vi "AlliGator Plot Fit Parameter 2 vs Parameter 1.vi"(7 "Lifetime Graph refnum":refnum<vi>, 8 "error in (no error)":errorcluster, 9 "Fit Parameter 2":T1, 10 "Fit Parameter 1":T1, 11 "Data Value Reference in":refnum<data-value>) -> (0 "error out":errorcluster, 3 "Data Value Reference out":refnum<data-value>, 4 "Message":string)   [LabVIEW 2021, in "AlliGator Decay Fit Parameter Map.lvlib"]
doc: "Creates scatter plot of selected parameter vs intensity for all ROIs and sends it to the <B>Lifetime & Other Parameters Graph</B>."
uses:
  AlliGator Decay Fit Parameter Map.lvlib
  Internal Variables/AlliGator Internal Variables v2.ctl
  <vilib>/vision/Image Controls.llb/IMAQ Image.ctl
  Internal Variables/AlliGator Gate Image Set.ctl
  Files/AlliGator FLI Dataset Type.ctl
  Files/AlliGator Data Series Type.ctl
  Dual-Channel Datasets/AlliGator Dataset Channel.ctl
  Settings/AlliGator Gate Arithmetic.ctl
  Source Image/AlliGator Displayed Image.ctl
  Image/Named ROI Description.ctl
  Phasor Graph/AlliGator Decay Metadata v3.ctl
  Decay Analysis/Decay Preprocessing/AlliGator Decay Background Subtraction Info.ctl
  Decay Analysis/Decay Preprocessing/AlliGator Baseline Subtraction Method.ctl
  Graphs/XY Graph/XY Graph Plot Shift Parameters.ctl
  Graphs/XY Graph/XY Graph Plot Shift Method.ctl
  Decay Analysis/Decay Preprocessing/AlliGator Decay Extrapolation Parameters.ctl
  Phasor/Calibration Phasor (m, phi).ctl
  Phasor/Phasor Reference Series.ctl
  Phasor/Phasor Calibration Map v2.ctl
  Phasor/Phasor (g, s).ctl
  Phasor Graph/AlliGator Raw Phasor Plot Data v5.ctl
  Phasor/Phasor Standard Deviation Options.ctl
  Phasor Plot/AlliGator Phasor Multi-Harmonic Data.ctl
  Phasor/Phasor Harmonic Data.ctl
  AlliGator Decay Fit Options & Parameters v4.ctl
  Fits/IRF(X)PSED/Decay Fit Options v4.ctl
  Fits/Decay Convolution/Decay Model.ctl
  Fits/Residual Type.ctl
  Fits/IRF(X)PSED/Fit Weights Type v2.ctl
  Fits/Non-linear Fitting Method v2.ctl
  Fits/Fit Calculation Method.ctl
  Fits/Non-linear Fitting Algorithm.ctl
  Decay Analysis/Decay Fit/AlliGator Decay Fit Parameter Constraints 2.ctl
  Fits/IRF(X)PSED/Decay Fit Parameters In List.ctl
  Fits/IRF(X)PSED/MLE Baseline Offset Type.ctl
  Decay Analysis/Decay Preprocessing/AlliGator Decay Preprocessing Parameters.ctl
  Fits/IRF(X)PSED/Decay Fit Parameters & Derived Quantities List v2.ctl
  Fits/IRF(X)PSED/Decay Fit Result Constraint.ctl
  AlliGator Parameter Maps Data.ctl
  Graphs/LabVIEW Plot Interpolation.ctl
  Graphs/Plot Point Style.ctl
  <userlib>/_OpenG.lib/array/array.llb/Filter 1D Array with Scalar (DBL)__ogtk.vi
  <userlib>/_OpenG.lib/array/array.llb/Delete Elements from 1D Array (DBL)__ogtk.vi
  <vilib>/Utility/error.llb/Error Cluster From Error Code.vi
  <vilib>/ErrorRing/Error Ring.xnode
  Files/AlliGator Files.lvlib
  Graphs/XY Graph/XY Graph Add-Ons.lvlib
  Graphs/Graphs.lvlib
  Image/Image.lvlib
  <userlib>/_OpenG.lib/array/array.llb/openg_array.lvlib
  Phasor/Phasor.lvlib
  Decay Analysis/Decay Preprocessing/AlliGator Decay Preprocessing.lvlib
  Phasor Graph/AlliGator Phasor Graph.lvlib
  Phasor Plot/AlliGator Phasor Plot.lvlib
  Source Image/AlliGator Source Image.lvlib
  Fits/Fits.lvlib
  Internal Variables/AlliGator Internal Variables.lvlib
  Decay Analysis/Decay Fit/AlliGator Decay Fit.lvlib
  Settings/AlliGator Settings.lvlib
  Dual-Channel Datasets/AlliGator Dual-Channel Datasets.lvlib
panel:
  in  "ROI idx (2147483647: all ROIs)":i32=2147483647
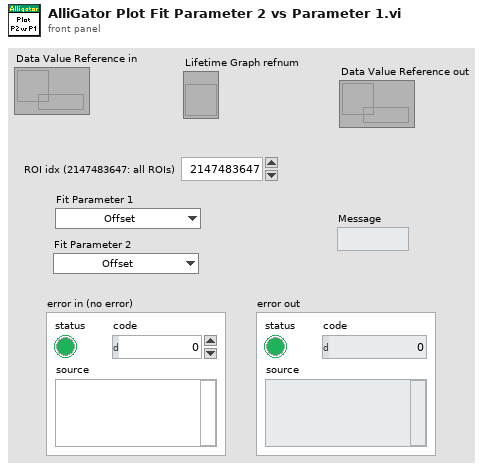
[diagram p1: front panel]
types:
  T1 = typedef "Fits.lvlib/Decay Fit Parameters & Derived Quantities List v2.ctl" = enum16{"Offset", "Baseline", "A_1", "tau_1", "A_2", "tau_2", "<tau>_a", "f1_a", "f2_a", "<tau>_i", "f1_i", "f2_i", "-", "R^2", "Chi^2"}
  T2 = typedef "Graphs.lvlib/Plot Point Style.ctl" = enum16{"not defined", "None", "Empty Circle", "Filled Circle", "Thick Circle", "Dotted Circle", "Empty Square", "Filled Square", "Thick Square", "Dotted Square", "Small Filled Square", "Dot", "Cross", "Tiny Cross", "Large X", "Small x", "Diamond", "Small Empty Square"}
  T3 = typedef "Graphs.lvlib/LabVIEW Plot Interpolation.ctl" = enum16{"Point (.)", "Stepwise Right (--.)", "Line + Point (\\. /)", "Stepwise Left (.--)", "Stepwise Centered (-.-)", "Stepwise Vertical (|.|)", "Line (-)", "Use Previous Plot's Style"}
  T4 = typedef "AlliGator Internal Variables.lvlib/AlliGator Internal Variables v2.ctl" = cluster{"----------------------------- Images -----------------------------":u8, "Displayed Image":T5, "White Light Image":T5, "Mask Image":T5, "ROI Mask Image":T5, "Current Dataset Images 1":T6, "Background Dataset Images 1":T6, "Current Dataset Images 2":T6, "Background Dataset Images 2":T6, "Current Dataset Arithmetic Images":T6, "Accumulated Dataset Images 1":T6, "Accumulated Dataset Images 2":T6, "Accumulated Dataset Arithmetic Images":T6, "----------------------------- File Paths -----------------------------":u8, "Phasor Plot Image":T5, "Decay Fit Parameter Map Image":T5, "Parameter Map Image":T5, "Single Data Point Path":path, "White Light Image Path":path, "Mask Image Path":path, "Time-Series Folder":path, "[Time-Series Paths]":path[], "----------------------------- FLI Dataset -----------------------------":u8, "Current Dataset":i32, "Single Dataset Type":T7, "Current Folder":string, "AlliGator Data Series Type":T8, "# Datasets":i32, "Dual-Channel Dataset":bool, "Selected Channel Name":string, "Dataset Channel":T9, "Channel Arithmetic":T10, "Dual-Channel Background Dataset":bool, "Background Channel":T9, "Dual-Channel Accumulated Dataset":bool, "Start Time":dbl, "[Time-Series Timestamps]":dbl[], "[Intensity Corrections]":dbl[], "Time Series Script":bool, "Type of Displayed Image":T11, "Gate Image Slide":u16, "# Gates":i32, "ROIs":T12[], "----------------------------- Decays -----------------------------":u8, "ROI Decay":cluster{"t Array":dbl[], "I Array":dbl[]}, "Valid Decay":bool, "Decay  Metadata":T14, "Reference Decay Plot Name":string, "Reference Decay":cluster{"t Array":dbl[], "I Array":dbl[]}, "Decay Shift Plot":cluster{"Time Stamps":dbl[], "Decay Shifts":dbl[]}, "[Decays Max Values]":sgl[], "[Decays Min Values]":sgl[], "----------------------------- Calibration -----------------------------":u8, "Calibration Phasor":T20, "Calibration Phasor Series":T21, "Phasor Calibration Map":T22, "Calibration Map MD5 Digest":string, "----------------------------- Phasor Graph -----------------------------":u8, "Last Raw Phasor":T23, "Last Calibrated Phasor":T23, "Last Calibrated Phasor SDV":T23, "Phasor Graph:Phasor Plot":cluster{"g Array":dbl[], "s Array":dbl[]}, "Phasor Graph:Phasor SDV Plot":cluster{"g Array":dbl[], "s Array":dbl[]}, "[Phasor Graph:Raw Phasor Plots]":T24[], "Phasor Plot locked to Ref 1":i32, "[Phasor Plot(s) locked to Ref 1]":i32[], "[Phasor Plot(s) locked to Ref 2]":i32[], "[Pixel Phasors]":T23[], "----------------------------- Phasor Plot -----------------------------":u8, "[[Sum Image]]":dbl[][], "[[CSG Phasors]]":csg[][], "[[Valid Pixel?]]":bool[][], "[[Phasor Ratios]]":dbl[][], "[[Average Lifetimes]]":dbl[][], "Amplitude Weighted Average Lifetime":bool, "I/m/phi Dataset":cluster{"I/m/phi Dataset?":bool, "Base Frequency":dbl[unit], "Harmonic Orders":u8[]}, "Multi Phasor Plot Data":T26, "----------------------------- Decay Fit Parameter Map -----------------------------":u8, "Decay Fit Options & Parameters":T28, "Fit Options: Decay Preprocessing Parameters":T39, "Fit Options: Reference Decay":cluster{"t Array":dbl[], "I Array":dbl[]}, "Is Full Image Parameters Map":bool, "Is Single-Pixels Parameters Map":bool, "NLSF Parameters Map X Resolution":i32, "NLSF Parameters Map Y Resolution":i32, "[Single Decay Fit Parameters]":dbl[], "Fit Model":T30, "[[Multiple Decays Fit Parameters]]":dbl[][], "[[Multiple Decays Fit Parameter SDVs]]":dbl[][], "[[IRFs]]":dbl[][], "[ROI Descriptors]":T13[], "IRF Array Time Axis":dbl[], "Decay Array Time Axis":dbl[], "[Decay Fit Parameter Names]":T1[], "[Decay Sum]":dbl[], "Array of Decay Fit Result Constraints":T40[], "Selected ROIs Array":bool[], "----------------------------- Parameter Maps -----------------------------":u8, "[Map Set Names]":string[], "[Parameter Maps]":T41[], "[[User-defined Quantities]]":dbl[][], "User-defined Quantity":string}
  T5 = typedef "IMAQ Image.ctl" = refnum<image>
  T6 = typedef "AlliGator Internal Variables.lvlib/AlliGator Gate Image Set.ctl" = cluster{"SGL Gate Images":T5[], "SGL Sum Image":T5, "SGL Max Image":T5, "SGL Min Image":T5}
  T7 = typedef "AlliGator Files.lvlib/AlliGator FLI Dataset Type.ctl" = enum16{"HDF5 FLI Dataset", "Gate Image Folder", ".sdt FLI Dataset (Becker & Hickl)", ".ptu FLI Dataset (PicoQuant)", "SS1 FLI Dataset", "SS2 FLI Dataset", "I/m/phi Dataset", ".bin FLI Dataset (PicoQuant Binned)", ".bin FLI Dataset (Piccolo Binned)", ".mat FLI Dataset"}
  T8 = typedef "AlliGator Files.lvlib/AlliGator Data Series Type.ctl" = enum16{"Not a Supported Series", "Gate Images Folder Series", "SwissSPAD 2 Dataset Series", "B&H FLI Dataset Series", "PicoQuant PTU FLI Dataset Series", "PicoQuant BIN FLI Dataset Series", "Piccolo hist BIN FLI Dataset Series", "HDF5 FLI Dataset Series"}
  T9 = typedef "AlliGator Dual-Channel Datasets.lvlib/AlliGator Dataset Channel.ctl" = enum16{"G2", "INT"}
  T10 = typedef "AlliGator Settings.lvlib/AlliGator Gate Arithmetic.ctl" = enum16{"None", "INT-G2", "G2/INT*<INT>", "(1 - G2/INT)*<INT>"}
  T11 = typedef "AlliGator Source Image.lvlib/AlliGator Displayed Image.ctl" = enum16{"Single Gate", "Sum of All Gates", "Max of All Gates", "Min of All Gates", "-", "White Ligth Image", "Mask Image"}
  T12 = typedef "Image.lvlib/Named ROI Description.ctl" = cluster{"ROI Descriptor":T13, "ROI Name":string, "Overlay Color":u32}
  T13 = typedef "ROI Descriptor" = cluster{"Global Rectangle":i32[], "Contours":cluster{"ID":enum32{"External", "Internal"}, "Type":u32, "Coordinates":i32[]}[]}
  T14 = typedef "AlliGator Phasor Graph.lvlib/AlliGator Decay Metadata v3.ctl" = cluster{"ROI Descriptor":T13, "ROI Center":cluster{"X":i32, "Y":i32}, "Decay Background Subtraction Info":T15, "Decay Reverted":bool, "Decay Smoothened":bool, "Decay Straightened":bool, "Fitted Tau (Decay Straightening)":dbl, "Decay Shift Parameters":T17, "Decay Shifted":bool, "Decay Extrapolated":bool, "Decay Extrapolation Parameters":T19, "Decay Normalized":bool, "Fold Decay":bool, "# Folds":u32}
  T15 = typedef "AlliGator Decay Preprocessing.lvlib/AlliGator Decay Background Subtraction Info.ctl" = cluster{"Laser Period":dbl[unit], "Gate Duration":dbl[unit], "Baseline Subtraction Method":T16, "Background Definition Range":cluster{"Min Gate":dbl[unit], "Max Gate":dbl[unit]}, "Total Intensity w/o Bkgd Subtraction":dbl, "Bkgd-subtracted Intensity (exp)":dbl, "# Data Points":i32, "Background/Gate":dbl, "Fitted Lifetime":dbl[unit], "Bkgd-subtracted Intensity (theo)":dbl}
  T16 = typedef "AlliGator Decay Preprocessing.lvlib/AlliGator Baseline Subtraction Method.ctl" = enum16{"Mean", "Min", "Square Gated Single-Exponential", "File", "Constant"}
  T17 = typedef "XY Graph Add-Ons.lvlib/XY Graph Plot Shift Parameters.ctl" = cluster{"Type":T18, "Shift":dbl[unit], "Threshold":dbl, "Rotate":bool}
  T18 = typedef "XY Graph Add-Ons.lvlib/XY Graph Plot Shift Method.ctl" = enum16{"Default", "CFD", "Threshold", "Cross-Correlation"}
  T19 = typedef "AlliGator Decay Preprocessing.lvlib/AlliGator Decay Extrapolation Parameters.ctl" = cluster{"Additional Points":u32, "Head Fraction":dbl, "Fitted Tau":dbl, "Use Periodicity":bool, "Use Cursors":bool, "Tail Fraction":dbl}
  T20 = typedef "Phasor.lvlib/Calibration Phasor (m, phi).ctl" = cluster{"m":dbl, "phi":dbl, "Phasor Frequency":dbl[unit], "Reference Lifetime":dbl[unit]}
  T21 = typedef "Phasor.lvlib/Phasor Reference Series.ctl" = cluster{"m Array":dbl[], "phi Array":dbl[], "Phasor Frequency":dbl[unit], "Calibration Lifetime":dbl[unit]}
  T22 = typedef "Phasor.lvlib/Phasor Calibration Map v2.ctl" = cluster{"Phasor Frequency":dbl[unit], "Calibration Lifetime":dbl[unit], "ROI Centers":cluster{"X":i32, "Y":i32}[], "ROI Descriptors":T13[], "Map Resolution X":i32, "Map Resolution Y":i32, "z Array":cdb[]}
  T23 = typedef "Phasor.lvlib/Phasor (g, s).ctl" = cluster{"g":dbl, "s":dbl}
  T24 = typedef "AlliGator Phasor Graph.lvlib/AlliGator Raw Phasor Plot Data v5.ctl" = cluster{"Phasor Plot Name":string, "Raw Phasor Plot":T23[], "Phasor Frequency":dbl[unit], "[Decay Metadata]":T14[], "Raw Phasor Plot SDV":T23[], "Phasor SDV Options":T25, "[Calibration Phasor]":T20[], "Intensity Array":dbl[]}
  T25 = typedef "Phasor.lvlib/Phasor Standard Deviation Options.ctl" = cluster{"Compute Estimated SDV":bool, "# Replicas":u32, "Use Estimated Average Phasor":bool}
  T26 = typedef "AlliGator Phasor Plot.lvlib/AlliGator Phasor Multi-Harmonic Data.ctl" = cluster{"Base Frequency":dbl[unit], "# Harmonics":u8, "Harmonic Orders":u8[], "Phasor Plot Settings Checksum":u64, "Phasor Harmonic Data Array":T27[]}
  T27 = typedef "Phasor.lvlib/Phasor Harmonic Data.ctl" = cluster{"Phasor Harmonic Name":string, "Phasor Plot Settings Checksum":u64, "Phasor Frequency":dbl[unit], "Base Frequency":dbl[unit], "Harmonic Order":u8, "Phasor Plot Parameters":string, "Phasor Array [[CSG]]":csg[][], "Dataset File Path":path}
  T28 = typedef "AlliGator Decay Fit Parameter Map.lvlib/AlliGator Decay Fit Options & Parameters v4.ctl" = cluster{"SYNC Period":dbl[unit], "Fit Options":T29, "Fit Parameter Constraints":T36[], "MLE Baseline Offset":dbl, "MLE Baseline Offset Type":T38}
  T29 = typedef "Fits.lvlib/Decay Fit Options v4.ctl" = cluster{"Show Fit Residuals":bool, "Fit Model":T30, "Residual Type":T31, "Max Decay Percentile":dbl, "Min Decay Percentile":dbl, "Show Full Decay":bool, "Weights":T32, "Fitting Method":T33, "Compute Parameter Uncertainties":bool, "Periodic Boundaries":bool, "Model Calculation":T34, "Period":dbl[unit], "Termination Criteria":cluster{"Max Iterations":i32, "Max Function Calls":i32, "Max Time":dbl[unit], "Function Tolerance":dbl, "Parameter Tolerance":dbl, "Gradient Tolerance":dbl, "Min Lambda":dbl, "Max Lambda":dbl, "Initial Tick Count":u32}, "Offset Resolution":dbl[unit], "Use Local IRF":bool, "Fitting Algorithm":T35, "Show Confidence Interval ":bool, "Confidence Level":dbl}
  T30 = typedef "Fits.lvlib/Decay Model.ctl" = enum16{"1-Exponential", "2-Exponentials"}
  T31 = typedef "Fits.lvlib/Residual Type.ctl" = enum16{"Standard", "Normalized", "Reduced"}
  T32 = typedef "Fits.lvlib/Fit Weights Type v2.ctl" = enum16{"Unweighted", "1/Variance (Neyman)", "1/Variance (Pearson)", "Best of All"}
  T33 = typedef "Fits.lvlib/Non-linear Fitting Method v2.ctl" = enum16{"Least Square", "Least Absolute Residual", "Bisquare", "MLE", "-", "Best of All"}
  T34 = typedef "Fits.lvlib/Fit Calculation Method.ctl" = enum16{"Simulation", "Convolution", "Integration"}
  T35 = typedef "Fits.lvlib/Non-linear Fitting Algorithm.ctl" = enum16{"Levenberg-Marquardt", "Trust-Region Dogleg"}
  T36 = typedef "AlliGator Decay Fit.lvlib/AlliGator Decay Fit Parameter Constraints 2.ctl" = cluster{"Fit Parameter":T37, "Min Value":dbl, "Max Value":dbl, "Global":bool, "Used":bool}
  T37 = typedef "Fits.lvlib/Decay Fit Parameters In List.ctl" = enum16{"Offset", "Baseline", "A_1", "tau_1", "A_2", "tau_2"}
  T38 = typedef "Fits.lvlib/MLE Baseline Offset Type.ctl" = enum32{"Absolute", "Percentage"}
  T39 = typedef "AlliGator Decay Preprocessing.lvlib/AlliGator Decay Preprocessing Parameters.ctl" = cluster{"Background Subtraction":bool, "Straighten Decay":bool, "Reverse Gates":bool, "1-Normalized Decay":bool, "Smoothen Decay":bool, "Smoothing Parameter":dbl, "Shift Decay":bool, "Decay Shift Parameters":T17, "Extrapolate Decay":bool, "Additional Points":u32, "Head Fraction":dbl, "Pixel-Normalize Decay":bool, "Use Periodicity":bool, "Use Cursors":bool, "Tail Fraction":dbl, "Use Decay Pre-Processing":bool, "Fold Decay":bool, "# Folds":u32, "[0-1]-Normalized Decay":bool}
  T40 = typedef "Fits.lvlib/Decay Fit Result Constraint.ctl" = cluster{"Fit Parameter":enum16{"Offset", "Baseline", "A_1", "tau_1", "A_2", "tau_2", "<tau>_a", "f1_a", "f2_a", "<tau>_i", "f1_i", "f2_i", "-", "R^2", "Chi^2", "Max Relative Residual", "<Residual ACF>", "Residual ACF SDV", "tau_2/tau_1"}, "Min Value":dbl, "Max Value":dbl, "Use Constraint":bool}
  T41 = typedef "AlliGator Decay Fit Parameter Map.lvlib/AlliGator Parameter Maps Data.ctl" = cluster{"Map Set Name":string, "[Parameter Names]":string[], "[[Parameters]]":dbl[][], "[[Parameter SDVs]]":dbl[][], "Decay Array Time Axis":dbl[], "[[IRFs]]":dbl[][], "IRF Array Time Axis":dbl[], "X Resolution":i32, "Y Resolution":i32, "Intensity Array":dbl[]}
  T42 = typedef "XY Graph Add-Ons.lvlib/XY Graph Refnum.ctl" = refnum<vi>
  T43 = cluster{"array w/ subset deleted":dbl[], "array w/ subset deleted":dbl[]}
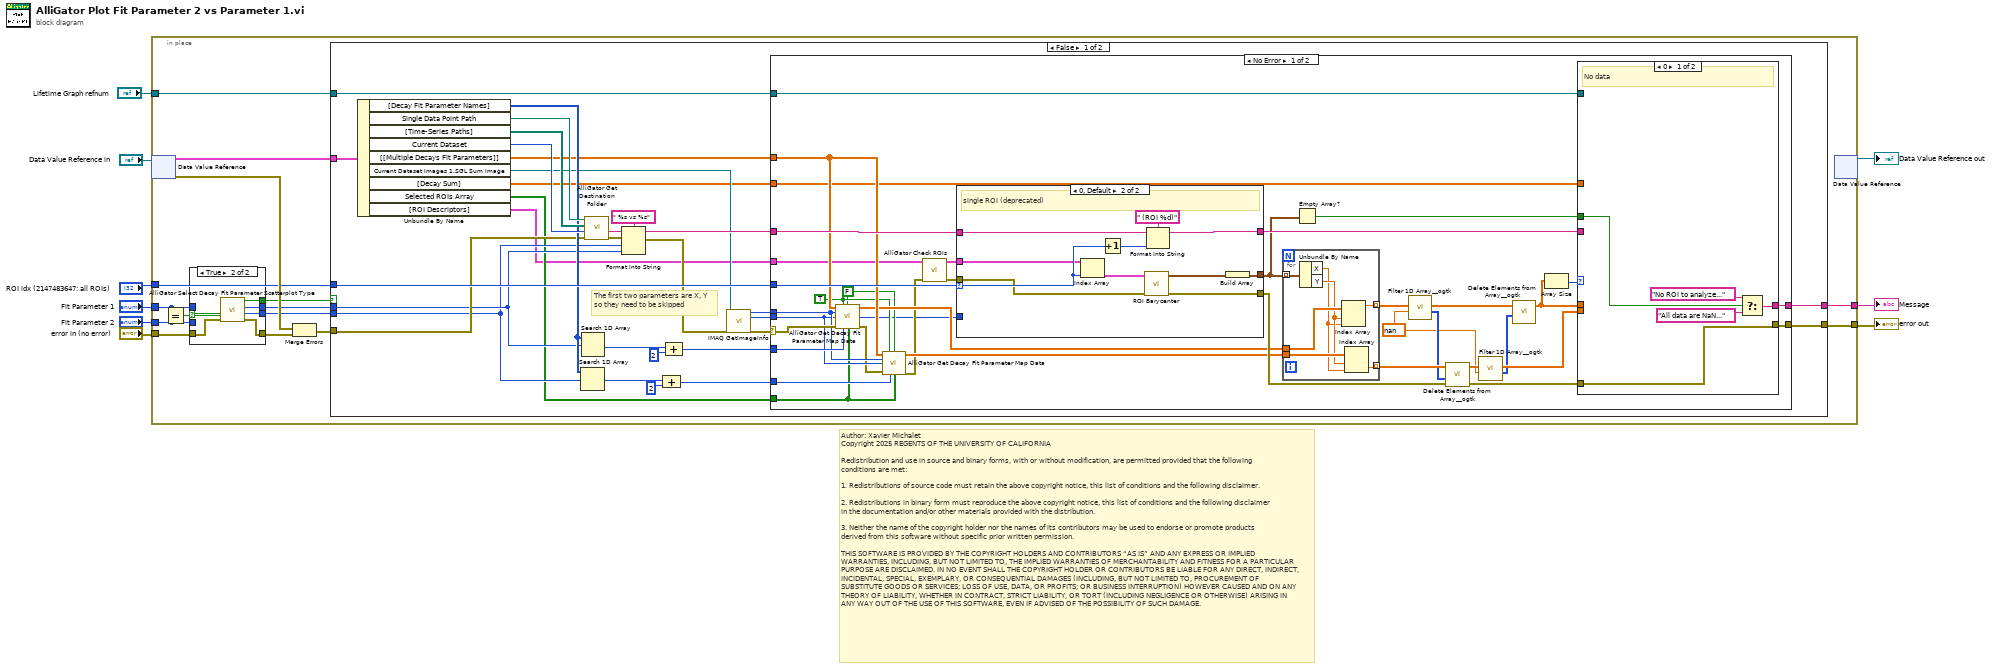
[diagram p0: block diagram]
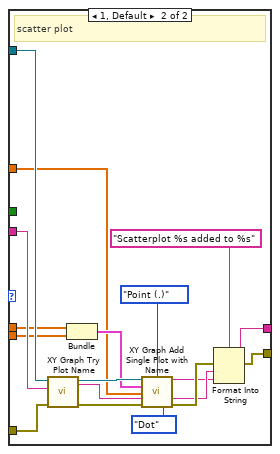
[diagram p2: hidden frame]
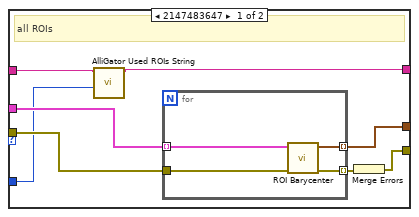
[diagram p3: hidden frame]
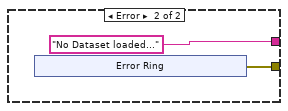
[diagram p4: hidden frame]
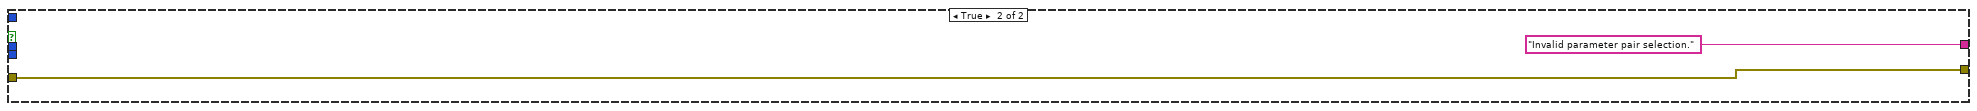
[diagram p5: hidden frame]
diagram:
  # "Author: Xavier Michalet\nCopyright 2025 REGENTS OF THE UNIVERSITY OF CALIFORNIA\n\nRedistribution and use in source and binary forms, with or without modification, are permitted provided that the following conditions are met:\n\n1. Redistributions of source code must retain the above copyright notice, this list of conditions and the following disclaimer.\n\n2. Redistributions in binary form must reproduce the above copyright notice, this list of conditions and the following disclaimer in the documentation and/or other materials provided with the distribution.\n\n3. Neither the name of the copyright holder nor the names of its contributors may be used to endorse or promote products derived from this software without specific prior written permission.\n\nTHIS SOFTWARE IS PROVIDED BY THE COPYRIGHT HOLDERS AND CONTRIBUTORS “AS IS” AND ANY EXPRESS OR IMPLIED WARRANTIES, INCLUDING, BUT NOT LIMITED TO, THE IMPLIED WARRANTIES OF MERCHANTABILITY AND FITNESS FOR A PARTICULAR PURPOSE ARE DISCLAIMED. IN NO EVENT SHALL THE COPYRIGHT HOLDER OR CONTRIBUTORS BE LIABLE FOR ANY DIRECT, INDIRECT, INCIDENTAL, SPECIAL, EXEMPLARY, OR CONSEQUENTIAL DAMAGES (INCLUDING, BUT NOT LIMITED TO, PROCUREMENT OF SUBSTITUTE GOODS OR SERVICES; LOSS OF USE, DATA, OR PROFITS; OR BUSINESS INTERRUPTION) HOWEVER CAUSED AND ON ANY THEORY OF LIABILITY, WHETHER IN CONTRACT, STRICT LIABILITY, OR TORT (INCLUDING NEGLIGENCE OR OTHERWISE) ARISING IN ANY WAY OUT OF THE USE OF THIS SOFTWARE, EVEN IF ADVISED OF THE POSSIBILITY OF SUCH DAMAGE."
  n1 = in-place {
    in-place-border: "Fit Parameter 1" -> [w17]
    in-place-border: "error in (no error)" -> [w13]
    in-place-border: [w22] -> w3
    in-place-border: "Lifetime Graph refnum" -> [w21]
    in-place-border: "ROI idx (2147483647: all ROIs)" -> [w20]
    in-place-border: [w19] -> w4
    in-place-border: "Fit Parameter 2" -> [w16]
    n2 = in-place-dvr #1("Data Value Reference in") -> (w24:T4, w23:errorcluster)
    n3 = Equal?(x=w17, y=w16) -> (x = y?=w18:bool)
    n4 = case shown="True" w18 {
      tunnel: w17 -> [w155 _]
      tunnel: w16 -> [w154 _]
      tunnel: [w155 w160] -> w15
      tunnel: [w154 w159] -> w14
      tunnel: [_ w158] -> w11
      tunnel: w13 -> [w153 w157]
      tunnel: [w153 w156] -> w12
      frame False {
      }
      frame True {
        n5 = call "AlliGator Select Decay Fit Parameter Scatterplot Type.vi"("Error In"=w157) -> ("Error Out"=w156:errorcluster, "Fit Parameter 2"=w159:T1, "Fit Parameter 1"=w160:T1, "Cancelled?"=w158:bool)  [unwired: 7 in]
      }
    }
    n6 = Merge Errors(w23, w12) -> (w10:errorcluster)
    n7 = case shown="False" w11 {
      tunnel: w24 -> [w55 _]
      tunnel: [w54 w152] -> w22
      tunnel: w21 -> [w53 _]
      tunnel: w20 -> [w52 _]
      tunnel: [w51 "Invalid parameter pair selection."] -> w19
      tunnel: w15 -> [w32 _]
      tunnel: w14 -> [w31 _]
      tunnel: w10 -> [w40 w152]
      frame False {
        # "The first two parameters are X, Y so they need to be skipped"
        n8 = Unbundle By Name(w55) -> ("[Decay Fit Parameter Names]"=w41:T1[], "Single Data Point Path"=w47:path, "[Time-Series Paths]"=w46:path[], "Current Dataset"=w45:i32, "[[Multiple Decays Fit Parameters]]"=w33:dbl[][], "Current Dataset Images 1.SGL Sum Image"=w39:T5, "[Decay Sum]"=w30:dbl[], "Selected ROIs Array"=w26:bool[], "[ROI Descriptors]"=w25:T13[])
        n9 = Search 1D Array(1D array=w41, element=w31) -> (index of element=w35:i32)  [unwired: 1 in]
        n10 = Search 1D Array(1D array=w41, element=w32) -> (index of element=w48:i32)  [unwired: 1 in]
        n11 = call "AlliGator Get Destination Folder.vi"("Error In"=w40, "Current Data Set (-1: single)"=w45, "Time-Series Paths"=w46, "Single Data Point Path"=w47) -> ("Error Out"=w43:errorcluster, "Data Point Name"=w50:string)  [unwired: 4 in, 2 out]
        n12 = Format Into String(format string=" %s vs %s", initial string=w50, error in=w43, w31, w32) -> (resulting string=w44:string, error out=w42:errorcluster)
        n13 = Compound Arithmetic op=ADD(w35, 2 ("value")) -> (w34:i32)
        n14 = Compound Arithmetic op=ADD(w48, 2 ("value")) -> (w38:i32)
        n15 = call "IMAQ GetImageInfo"("error in (no error)"=w42, "Image"=w39) -> ("error out"=w29:errorcluster, "Y Resolution"=w27:i32, "X Resolution"=w28:i32)  [unwired: 2 in, 5 out]
        n16 = case shown="No Error" w29 {
          selector: w29 -> [w78 _]
          tunnel: [w91 w145] -> w54
          tunnel: w53 -> [w90 _]
          tunnel: w52 -> [w89 _]
          tunnel: [w88 "No Dataset loaded..."] -> w51
          tunnel: w44 -> [w87 _]
          tunnel: w38 -> [w86 _]
          tunnel: w34 -> [w83 _]
          tunnel: w33 -> [w81 _]
          tunnel: w30 -> [w80 _]
          tunnel: w28 -> [w77 _]
          tunnel: w27 -> [w76 _]
          tunnel: w26 -> [w71 _]
          tunnel: w25 -> [w70 _]
          frame No Error {
            w61 = nan ("items to filter")
            w72 = FALSE ("Output ROI centers?")
            w73 = TRUE ("Compute Decay Fit Parameter Map")
            n17 = call "AlliGator Get Decay Fit Parameter Map Data.vi"("Multiple Decays Fit Parameters"=w81, "Compute Decay Fit Parameter Map"=w73, "Output ROI centers?"=w72, "X Resolution"=w77, "Y Resolution"=w76, "Error In"=w78, "Map index"=w86, "Selected ROI Array"=w71) -> ("Map Data (V x H)"=w79:dbl[][], "# Filtered ROIs"=w66:i32, "Error Out"=w75:errorcluster)  [unwired: 3 in, 2 out]
            n18 = call "AlliGator Get Decay Fit Parameter Map Data.vi"("Multiple Decays Fit Parameters"=w81, "Compute Decay Fit Parameter Map"=w73, "Output ROI centers?"=w72, "X Resolution"=w77, "Y Resolution"=w76, "Error In"=w75, "Map index"=w83, "Selected ROI Array"=w71) -> ("Map Data (V x H)"=w74:dbl[][], "Error Out"=w69:errorcluster)  [unwired: 3 in, 3 out]
            n19 = call "AlliGator Check ROIs.vi"("error in (no error)"=w69, "[ROI Descriptors] in"=w70) -> ("error out"=w68:errorcluster, "[ROI Descriptors] out"=w67:T13[])  [unwired: 8 in]
            n20 = case shown="0, Default" w89 {
              selector: w89 -> [_ w141]
              tunnel: [w129 w136] -> w82
              tunnel: w87 -> [w124 w144]
              tunnel: [w123 w142] -> w84
              tunnel: [w128 w138] -> w57
              tunnel: w68 -> [w125 w134]
              tunnel: w67 -> [w126 w135]
              tunnel: w66 -> [w122 _]
              frame 2147483647 {
                # "all ROIs"
                n21 = call "AlliGator Used ROIs String.vi"("# Filtered ROIs"=w122, "String in"=w124) -> ("String out"=w123:string)  [unwired: 9 in]
                n22 = for {
                  tunnel: w126 -> [w133] mode=indexing
                  tunnel: w125 -> [w131]
                  tunnel: [w132] -> w128 mode=indexing
                  tunnel: [w130] -> w127 mode=indexing
                  n23 = call "ROI Barycenter.vi"("Error In"=w131, "ROI Descriptor in"=w133) -> ("Error Out"=w130:errorcluster, "ROI Center"=w132:cluster{"X":dbl, "Y":dbl})  [unwired: 7 in, 1 out]
                }
                n24 = Merge Errors(w127) -> (w129:errorcluster)
              }
              frame 0, Default {
                # "single ROI (deprecated)"
                n25 = Index Array(array=w135, index=w141) -> (element=w137:T13)
                n26 = Increment(x=w141) -> (x+1=w140:i32)
                n27 = call "ROI Barycenter.vi"("Error In"=w134, "ROI Descriptor in"=w137) -> ("Error Out"=w136:errorcluster, "ROI Center"=w139:cluster{"X":dbl, "Y":dbl})  [unwired: 7 in, 1 out]
                n28 = Format Into String(format string=" (ROI %d)", initial string=w144, w140) -> (resulting string=w142:string)  [unwired: 1 in, 1 out]
                n29 = Build Array(w139) -> (w138:cluster{"X":dbl, "Y":dbl}[])
              }
            }
            n30 = for {
              tunnel: w79 -> [w121]
              tunnel: [w120] -> w65 mode=indexing
              tunnel: w57 -> [w119] mode=indexing
              tunnel: w74 -> [w118]
              tunnel: [w116] -> w64 mode=indexing
              n31 = Unbundle By Name(w119) -> ("X"=w115:dbl, "Y"=w117:dbl)
              n32 = Index Array(array=w121, index (row)=w117, index (col)=w115) -> (element=w120:dbl)
              n33 = Index Array(array=w118, index (row)=w117, index (col)=w115) -> (element=w116:dbl)
            }
            n34 = Empty Array?(array=w57) -> (empty?=w56:bool)
            n35 = call-poly <userlib>:"Filter 1D Array__ogtk.vi"("items to filter"=w61, "array"=w65) -> ("filtered item indices"=w62:i32[], "filtered array"=w60:dbl[])  [unwired: 4 in]
            n36 = call-poly <userlib>:"Delete Elements from Array__ogtk.vi"("indices"=w62, "array"=w64) -> ("array w/ subset deleted"=w63:dbl[])  [unwired: 8 in, 1 out]
            n37 = call-poly <userlib>:"Filter 1D Array__ogtk.vi"("items to filter"=w61, "array"=w63) -> ("filtered item indices"=w58:i32[])  [unwired: 4 in, 1 out]
            n38 = call-poly <userlib>:"Delete Elements from Array__ogtk.vi"("indices"=w58, "array"=w60) -> ("array w/ subset deleted"=w59:dbl[])  [unwired: 8 in, 1 out]
            n39 = Array Size(array=w59) -> (size(s)=w85:i32)
            n40 = case shown="0" w85 {
              tunnel: w84 -> [_ w114]
              tunnel: w90 -> [_ w113]
              tunnel: [w96 w108] -> w91
              tunnel: w59 -> [_ w100]
              tunnel: [w94 w103] -> w88
              tunnel: w63 -> [_ w99]
              tunnel: w82 -> [w96 w98]
              tunnel: w80 -> [_ w97]
              tunnel: w56 -> [w93 _]
              frame 0 {
                # "No data"
                n41 = Select(t="No ROI to analyze...", s=w93, f="All data are NaN...") -> (s? t:f=w94:string)
              }
              frame 1, Default {
                # "scatter plot"
                n42 = call "XY Graph Try Plot Name.vi"("Error In"=w98, "Plot Name in"=w114, "XY Graph Refnum"=w113) -> ("Error Out"=w112:errorcluster, "Plot Name out"=w111:string, "XY Graph Refnum"=w110:T42)  [unwired: 5 in, 1 out]
                n43 = Bundle("array w/ subset deleted"=w100, "array w/ subset deleted"=w99) -> (w104:T43)  [unwired: 1 in]
                n44 = call "XY Graph Add Single Plot with Name.vi"("XYGraph Ref in"=w110, "Plot Interpolation (Previous Plot's Style)"=LabVIEW_Plot_Interpolation."Point (.)", "Plot"=w104, "Plot Metadata"=w97, "Plot Name (\"Plot\")"=w111, "error in (no error)"=w112, "Point Style (Dot)"=Plot_Point_Style."Dot") -> ("XY Graph Caption (or Label)"=w106:string, "Plot Name"=w107:string, "error out"=w109:errorcluster)  [unwired: 5 in, 1 out]
                n45 = Format Into String(format string="Scatterplot %s added to %s", error in=w109, w107, w106) -> (resulting string=w103:string, error out=w108:errorcluster)  [unwired: 1 in]
              }
            }
          }
          frame Error {
            n46 = xnode "Error Ring"() -> ("error out"=w145:errorcluster)
          }
        }
      }
      frame True {
      }
    }
    n47 = in-place-dvr #1() -> (→"Data Value Reference out":refnum<data-value>)  [unwired: 1 in, 1 out]
  }
  "error out" <- w3
  "Message" <- w4
